vi "Limit Switch.vi"(1 "Input":bool) -> (0 "Output":dbl)   [LabVIEW 2013]
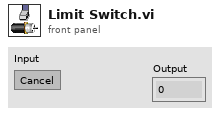
[diagram p1: front panel]
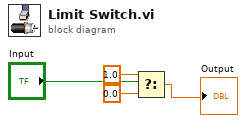
[diagram p0: block diagram]
diagram:
  n1 = Select(t=1.0, s="Input", f=0.0) -> (s? t:f=→"Output":dbl)
